vi "Lift Safety.vi"(11 "Operation States":T2) -> (3 "Operation States":T2)   [LabVIEW 2014]
uses:
  <vilib>/Rock Robotics/WPI/Solenoid/WPI_SolenoidValue.ctl
  <vilib>/Rock Robotics/Network Tables/SD Write Boolean.vi
  Robot Global Data.vi
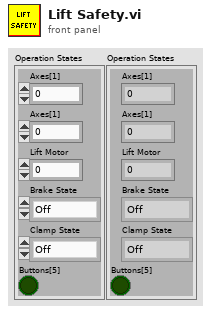
[diagram p1: front panel]
types:
  T1 = typedef "WPI_SolenoidValue.ctl" = enum16{"Off", "On", "Forward", "Reverse"}
  T2 = cluster{"Axes[1]":dbl, "Axes[1]":dbl, "Lift Motor":dbl, "Brake State":T1, "Clamp State":T1, "Buttons[5]":bool}
  T3 = typedef "WPI_SwitchDevRef.ctl" = cluster{"DevStatus":errorcluster, "DIO Channel":T4, "Controller":T5, "CntIndex":T6, "Normally Closed":bool}
  T4 = typedef "FPGA_DIOChannel.ctl" = enum8{"DIO 0", "DIO 1", "DIO 2", "DIO 3", "DIO 4", "DIO 5", "DIO 6", "DIO 7", "DIO 8", "DIO 9", "DIO MXP 0", "DIO MXP 1", "DIO MXP 2", "DIO MXP 3", "DIO MXP 4", "DIO MXP 5", "DIO MXP 6", "DIO MXP 7", "DIO MXP 8", "DIO MXP 9", "DIO MXP 10", "DIO MXP 11", "DIO MXP 12", "DIO MXP 13", "DIO MXP 14", "DIO MXP 15", "Invalid"}
  T5 = typedef "FPGA_TypedefDigitalModule.ctl" = enum16{"Controller 1"}
  T6 = typedef "FPGA_CounterCtrSystemIndex.ctl" = enum8{"Ctr 0", "Ctr 1", "Ctr 2", "Ctr 3", "Ctr 4", "Ctr 5", "Ctr 6", "Ctr 7", "Invalid"}
  T7 = enum16{"None", "Top Setpoint", "Bottom Setpoint", "Lower Setpoint", "Mid Setpoint"}
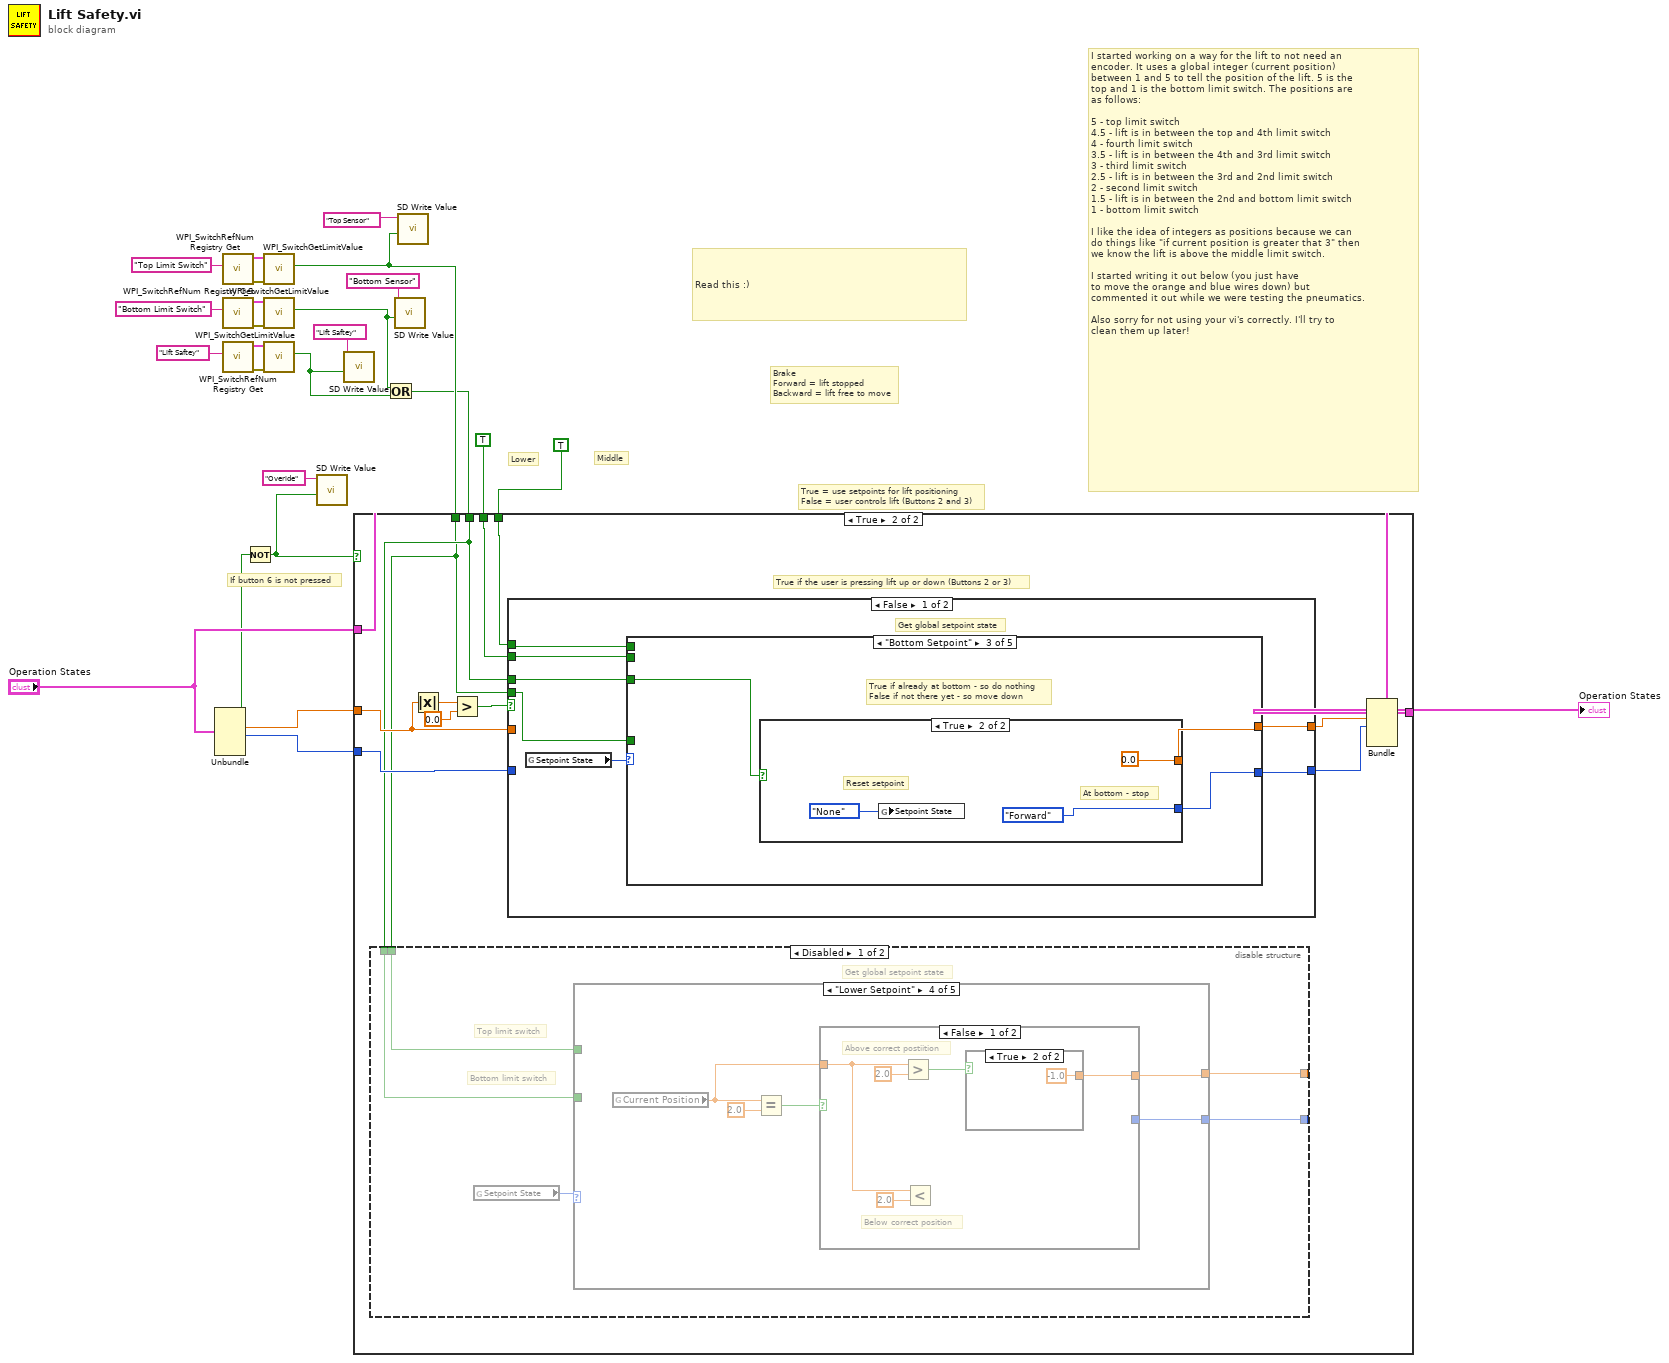
[diagram p0: block diagram]
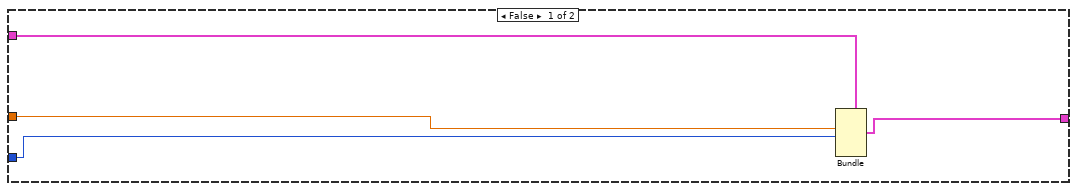
[diagram p2: hidden frame]
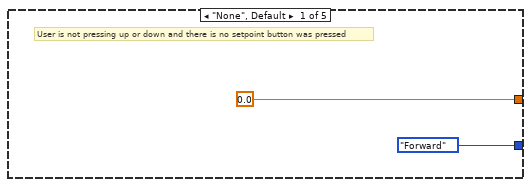
[diagram p3: hidden frame]
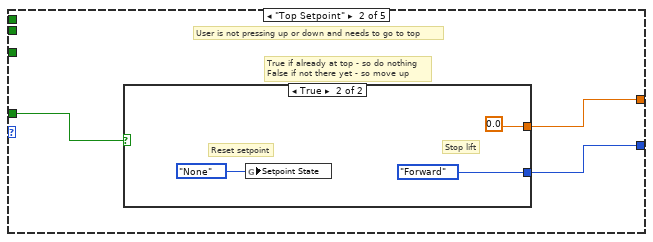
[diagram p4: hidden frame]
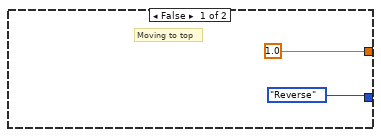
[diagram p5: hidden frame]
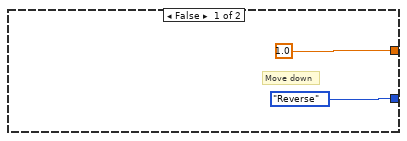
[diagram p6: hidden frame]
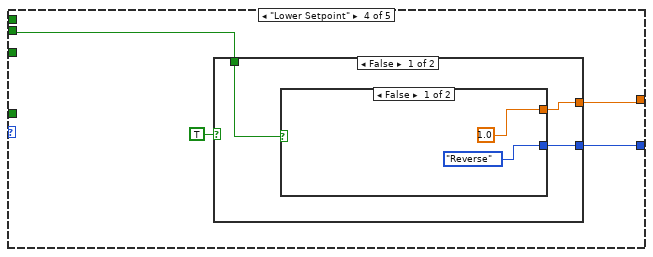
[diagram p7: hidden frame]
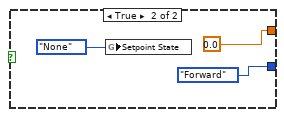
[diagram p8: hidden frame]
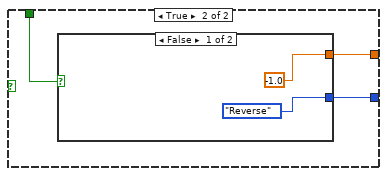
[diagram p9: hidden frame]
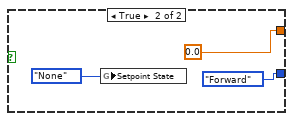
[diagram p10: hidden frame]
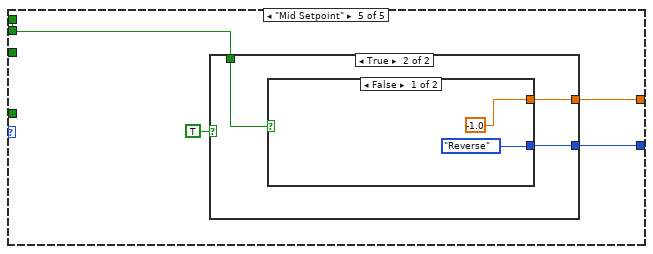
[diagram p11: hidden frame]
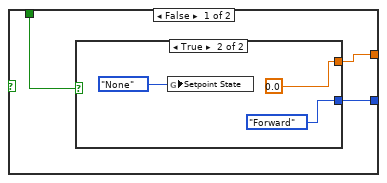
[diagram p12: hidden frame]
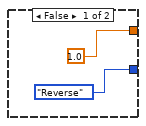
[diagram p13: hidden frame]
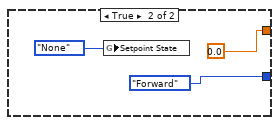
[diagram p14: hidden frame]
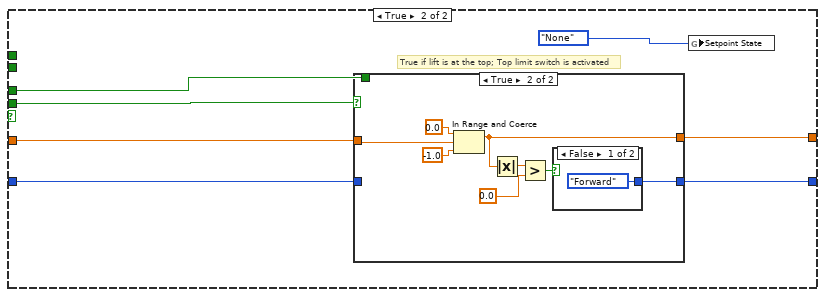
[diagram p15: hidden frame]
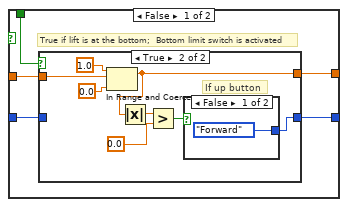
[diagram p16: hidden frame]
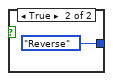
[diagram p18: hidden frame]
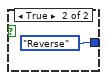
[diagram p19: hidden frame]
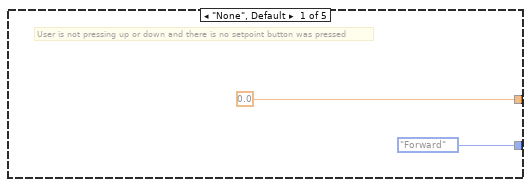
[diagram p20: hidden frame]
diagram:
  # "Read this :)"
  # "I started working on a way for the lift to not need an\nencoder. It uses a global integer (current position) \nbetween 1 and 5 to tell the position of the lift. 5 is the\ntop and 1 is the bottom limit switch. The positions are \nas follows:\n\n5 - top limit switch \n4.5 - lift is in between the top and 4th limit switch\n4 - fourth limit switch\n3.5 - lift is in between the 4th and 3rd limit switch\n3 - third limit switch\n2.5 - lift is in between the 3rd and 2nd limit switch\n2 - second limit switch\n1.5 - lift is in between the 2nd and bottom limit switch\n1 - bottom limit switch\n\nI like the idea of integers as positions because we can \ndo things like \"if current position is greater that 3\" then\nwe know the lift is above the middle limit switch.\n\nI started writing it out below (you just have \nto move the orange and blue wires down) but \ncommented it out while we were testing the pneumatics.\n\nAlso sorry for not using your vi's correctly. I'll try to \nclean them up later!"
  # "If button 6 is not pressed"
  # "Brake\nForward = lift stopped\nBackward = lift free to move"
  # "True = use setpoints for lift positioning\nFalse = user controls lift (Buttons 2 and 3)"
  # "Middle"
  # "Lower"
  n1 = Unbundle("Operation States") -> ("Lift Motor"=w24:dbl, "Brake State"=w25:T1, "Buttons[5]"=w4:bool)  [unwired: 3 out]
  n2 = call <vilib>:"WPI_SwitchRefNum Registry Get.vi"("refnum name"="Top Limit Switch") -> ("error out"=w11:errorcluster, "SwitchDevRef"=w12:T3)  [unwired: 9 in]
  n3 = call <vilib>:"WPI_SwitchRefNum Registry Get.vi"("refnum name"="Bottom Limit Switch") -> ("error out"=w13:errorcluster, "SwitchDevRef"=w14:T3)  [unwired: 9 in]
  n4 = call <vilib>:"WPI_SwitchRefNum Registry Get.vi"("refnum name"="Lift Saftey") -> ("error out"=w17:errorcluster, "SwitchDevRef"=w18:T3)  [unwired: 9 in]
  n5 = Not(x=w4) -> (.not. x?=w3:bool)
  n6 = call <vilib>:"WPI_SwitchGetLimitValue.vi"("error in (no error)"=w11, "SwitchDevRef"=w12) -> ("Switch Pressed"=w2:bool)  [unwired: 7 in, 2 out]
  n7 = call <vilib>:"WPI_SwitchGetLimitValue.vi"("error in (no error)"=w13, "SwitchDevRef"=w14) -> ("Switch Pressed"=w19:bool)  [unwired: 7 in, 2 out]
  n8 = call <vilib>:"WPI_SwitchGetLimitValue.vi"("error in (no error)"=w17, "SwitchDevRef"=w18) -> ("Switch Pressed"=w21:bool)  [unwired: 7 in, 2 out]
  n9 = call-poly <vilib>:"SD Write Value.vi"("Boolean"=w3, "Name"="Overide") -> ()  [unwired: 8 in, 2 out]
  n10 = call-poly <vilib>:"SD Write Value.vi"("Boolean"=w21, "Name"="Lift Saftey") -> ()  [unwired: 8 in, 2 out]
  n11 = Or(x=w19, y=w21) -> (x .or. y?=w1:bool)
  n12 = case shown="True" w3 {
    tunnel: "Operation States" -> [w29 w40]
    tunnel: [w26 w42] -> w5
    tunnel: w24 -> [w28 w39]
    tunnel: w25 -> [w27 w41]
    tunnel: w1 -> [_ w36]
    tunnel: w2 -> [_ w35]
    tunnel: TRUE -> [_ w38]
    tunnel: TRUE -> [_ w37]
    frame False {
      n13 = Bundle(cluster=w29, "Lift Motor"=w28, "Brake State"=w27) -> (w26:T2)  [unwired: 4 in]
    }
    frame True {
      # "True if the user is pressing lift up or down (Buttons 2 or 3)"
      n14 = disable-structure shown="Disabled" {
        disable-tunnel: w36 -> [w145 _]
        disable-tunnel: w35 -> [w144 _]
        disable-tunnel: [w143 _] -> _
        disable-tunnel: [w142 _] -> _
        frame Disabled {
          # "Top limit switch"
          # "Bottom limit switch"
          # "Get global setpoint state"
          n15 = global read "Robot Global Data.vi" "Setpoint State"() -> (w146:T7)
          n16 = case shown="\"Lower Setpoint\"" w146 {
            tunnel: [0.0 w151 w159 w167 w181] -> w143
            tunnel: [WPI_SolenoidValue."Forward" ("Brake State") w150 w158 w166 w180] -> w142
            tunnel: w145 -> [_ _ w157 _ _]
            tunnel: w144 -> [_ w149 _ _ _]
            frame "None", Default {
              # "User is not pressing up or down and there is no setpoint button was pressed"
            }
            frame "Top Setpoint" {
              # "True if already at top - so do nothing\nFalse if not there yet - so move up"
              # "User is not pressing up or down and needs to go to top"
              n17 = case shown="True" w149 {
                tunnel: [1.0 0.0] -> w151
                tunnel: [WPI_SolenoidValue."Reverse" ("Brake State") WPI_SolenoidValue."Forward" ("Brake State")] -> w150
                frame False {
                  # "Moving to top"
                }
                frame True {
                  # "Stop lift"
                  # "Reset setpoint"
                  n18 = global write "Robot Global Data.vi" "Setpoint State"(T7."None") -> ()
                }
              }
            }
            frame "Bottom Setpoint" {
              # "True if already at bottom - so do nothing\nFalse if not there yet - so move down"
              n19 = case shown="True" w157 {
                tunnel: [1.0 0.0] -> w159
                tunnel: [WPI_SolenoidValue."Reverse" ("Brake State") WPI_SolenoidValue."Forward" ("Brake State")] -> w158
                frame False {
                  # "Move down"
                }
                frame True {
                  # "At bottom - stop"
                  # "Reset setpoint"
                  n20 = global write "Robot Global Data.vi" "Setpoint State"(T7."None") -> ()
                }
              }
            }
            frame "Lower Setpoint" {
              n21 = global read "Robot Global Data.vi" "Current Position"() -> (w165:dbl)
              n22 = Equal?(x=w165, y=2.0) -> (x = y?=w168:bool)
              n23 = case shown="False" w168 {
                tunnel: [w170 0.0] -> w167
                tunnel: [_ WPI_SolenoidValue."Reverse" ("Brake State")] -> w166
                tunnel: w165 -> [w173 _]
                frame False {
                  # "Below correct position"
                  # "Above correct postiition"
                  n24 = Greater?(x=w173, y=2.0) -> (0:w171:bool)
                  n25 = Less?(x=w173, y=2.0) -> ()  [unwired: 1 out]
                  n26 = case shown="True" w171 {
                    tunnel: [_ -1.0] -> w170
                    frame False {
                    }
                    frame True {
                    }
                  }
                }
                frame True {
                  # "Reset setpoint"
                  n27 = global write "Robot Global Data.vi" "Setpoint State"(T7."None") -> ()
                }
              }
            }
            frame "Mid Setpoint" {
              n28 = case shown="True" TRUE {
                tunnel: [w183 w190] -> w181
                tunnel: [w182 w189] -> w180
                frame False {
                  n29 = case shown="True" {
                    selector: _ -> [_ _]
                    tunnel: [1.0 0.0] -> w183
                    tunnel: [WPI_SolenoidValue."Reverse" ("Brake State") WPI_SolenoidValue."Forward" ("Brake State")] -> w182
                    frame False {
                    }
                    frame True {
                      n30 = global write "Robot Global Data.vi" "Setpoint State"(T7."None") -> ()
                    }
                  }
                }
                frame True {
                  n31 = case shown="False" {
                    selector: _ -> [_ _]
                    tunnel: [-1.0 0.0] -> w190
                    tunnel: [WPI_SolenoidValue."Reverse" ("Brake State") WPI_SolenoidValue."Forward" ("Brake State")] -> w189
                    frame False {
                    }
                    frame True {
                      n32 = global write "Robot Global Data.vi" "Setpoint State"(T7."None") -> ()
                    }
                  }
                }
              }
            }
          }
        }
        frame Enabled {
        }
      }
      n33 = Absolute Value(x=w39) -> (abs(x)=w34:dbl)
      n34 = Greater?(x=w34, y=0.0) -> (0:w32:bool)
      n35 = case shown="False" w32 {
        tunnel: [w49 w114] -> w31
        tunnel: w36 -> [w43 w113]
        tunnel: [w46 w112] -> w30
        tunnel: w35 -> [w44 w111]
        tunnel: w39 -> [_ w110]
        tunnel: w41 -> [_ w109]
        tunnel: w38 -> [w48 _]
        tunnel: w37 -> [w47 _]
        frame False {
          # "Get global setpoint state"
          n36 = global read "Robot Global Data.vi" "Setpoint State"() -> (w45:T7)
          n37 = case shown="\"Bottom Setpoint\"" w45 {
            tunnel: [0.0 w54 w62 w71 w91] -> w49
            tunnel: w48 -> [_ _ _ _ w90]
            tunnel: w47 -> [_ _ _ w69 _]
            tunnel: [WPI_SolenoidValue."Forward" ("Brake State") w53 w61 w70 w89] -> w46
            tunnel: w44 -> [_ w52 _ _ _]
            tunnel: w43 -> [_ _ w60 _ _]
            frame "None", Default {
              # "User is not pressing up or down and there is no setpoint button was pressed"
            }
            frame "Top Setpoint" {
              # "True if already at top - so do nothing\nFalse if not there yet - so move up"
              # "User is not pressing up or down and needs to go to top"
              n38 = case shown="True" w52 {
                tunnel: [1.0 0.0] -> w54
                tunnel: [WPI_SolenoidValue."Reverse" ("Brake State") WPI_SolenoidValue."Forward" ("Brake State")] -> w53
                frame False {
                  # "Moving to top"
                }
                frame True {
                  # "Stop lift"
                  # "Reset setpoint"
                  n39 = global write "Robot Global Data.vi" "Setpoint State"(T7."None") -> ()
                }
              }
            }
            frame "Bottom Setpoint" {
              # "True if already at bottom - so do nothing\nFalse if not there yet - so move down"
              n40 = case shown="True" w60 {
                tunnel: [1.0 0.0] -> w62
                tunnel: [WPI_SolenoidValue."Reverse" ("Brake State") WPI_SolenoidValue."Forward" ("Brake State")] -> w61
                frame False {
                  # "Move down"
                }
                frame True {
                  # "At bottom - stop"
                  # "Reset setpoint"
                  n41 = global write "Robot Global Data.vi" "Setpoint State"(T7."None") -> ()
                }
              }
            }
            frame "Lower Setpoint" {
              n42 = case shown="False" TRUE {
                tunnel: [w73 w82] -> w71
                tunnel: w69 -> [w74 w81]
                tunnel: [w72 w80] -> w70
                frame False {
                  n43 = case shown="False" w74 {
                    tunnel: [1.0 0.0] -> w73
                    tunnel: [WPI_SolenoidValue."Reverse" ("Brake State") WPI_SolenoidValue."Forward" ("Brake State")] -> w72
                    frame False {
                    }
                    frame True {
                      n44 = global write "Robot Global Data.vi" "Setpoint State"(T7."None") -> ()
                    }
                  }
                }
                frame True {
                  n45 = case shown="False" w81 {
                    tunnel: [-1.0 0.0] -> w82
                    tunnel: [WPI_SolenoidValue."Reverse" ("Brake State") WPI_SolenoidValue."Forward" ("Brake State")] -> w80
                    frame False {
                    }
                    frame True {
                      n46 = global write "Robot Global Data.vi" "Setpoint State"(T7."None") -> ()
                    }
                  }
                }
              }
            }
            frame "Mid Setpoint" {
              n47 = case shown="True" TRUE {
                tunnel: [w93 w102] -> w91
                tunnel: w90 -> [w94 w101]
                tunnel: [w92 w100] -> w89
                frame False {
                  n48 = case shown="True" w94 {
                    tunnel: [1.0 0.0] -> w93
                    tunnel: [WPI_SolenoidValue."Reverse" ("Brake State") WPI_SolenoidValue."Forward" ("Brake State")] -> w92
                    frame False {
                    }
                    frame True {
                      n49 = global write "Robot Global Data.vi" "Setpoint State"(T7."None") -> ()
                    }
                  }
                }
                frame True {
                  n50 = case shown="False" w101 {
                    tunnel: [-1.0 0.0] -> w102
                    tunnel: [WPI_SolenoidValue."Reverse" ("Brake State") WPI_SolenoidValue."Forward" ("Brake State")] -> w100
                    frame False {
                    }
                    frame True {
                      n51 = global write "Robot Global Data.vi" "Setpoint State"(T7."None") -> ()
                    }
                  }
                }
              }
            }
          }
        }
        frame True {
          # "True if lift is at the top; Top limit switch is activated"
          n52 = case shown="True" w111 {
            tunnel: w110 -> [w118 w137]
            tunnel: w113 -> [w119 _]
            tunnel: [w117 w136] -> w114
            tunnel: [w116 w132] -> w112
            tunnel: w109 -> [w115 _]
            frame False {
              # "True if lift is at the bottom;  Bottom limit switch is activated"
              n53 = case shown="True" w119 {
                tunnel: w118 -> [w120 w127]
                tunnel: [w120 w122] -> w117
                tunnel: [w121 w126] -> w116
                tunnel: w115 -> [w121 _]
                frame False {
                  # "Lift is stopped; Always 0"
                }
                frame True {
                  # "If up button"
                  n54 = In Range and Coerce(upper limit=1.0, x=w127, lower limit=0.0) -> (coerced(x)=w122:dbl)  [unwired: 1 out]
                  n55 = Absolute Value(x=w122) -> (abs(x)=w125:dbl)
                  n56 = Greater?(x=w125, y=0.0) -> (0:w123:bool)
                  n57 = case shown="False" w123 {
                    tunnel: [WPI_SolenoidValue."Forward" ("Brake State") WPI_SolenoidValue."Reverse" ("Brake State")] -> w126
                    frame False {
                    }
                    frame True {
                    }
                  }
                }
              }
            }
            frame True {
              n58 = In Range and Coerce(upper limit=0.0, x=w137, lower limit=-1.0) -> (coerced(x)=w136:dbl)  [unwired: 1 out]
              n59 = Absolute Value(x=w136) -> (abs(x)=w135:dbl)
              n60 = Greater?(x=w135, y=0.0) -> (0:w133:bool)
              n61 = case shown="False" w133 {
                tunnel: [WPI_SolenoidValue."Forward" ("Brake State") WPI_SolenoidValue."Reverse" ("Brake State")] -> w132
                frame False {
                }
                frame True {
                }
              }
            }
          }
          n62 = global write "Robot Global Data.vi" "Setpoint State"(T7."None") -> ()
        }
      }
      n63 = Bundle(cluster=w40, "Lift Motor"=w31, "Brake State"=w30) -> (w42:T2)  [unwired: 4 in]
    }
  }
  "Operation States" <- w5
  n64 = call-poly <vilib>:"SD Write Value.vi"("Boolean"=w19, "Name"="Bottom Sensor") -> ()  [unwired: 8 in, 2 out]
  n65 = call-poly <vilib>:"SD Write Value.vi"("Boolean"=w2, "Name"="Top Sensor") -> ()  [unwired: 8 in, 2 out]
